vi "parsePlayInfo.vi"(7 "action":T3, 11 "variantInfo":variant) -> (3 "editArray":T1)   [LabVIEW 2014]
uses:
  typeDefs/parseAction.ctl
  typeDefs/editControl.ctl
  typeDefs/variantFlat.ctl
  typeDefs/labelInfo.ctl
  typeDefs/poiCommand.ctl
  typeDefs/jumpTpInfo.ctl
  typeDefs/syncInfo.ctl
  typeDefs/editViewPlay.ctl
panel:
  out "CODES":i32[][](array[numeric])
  out "Info":string
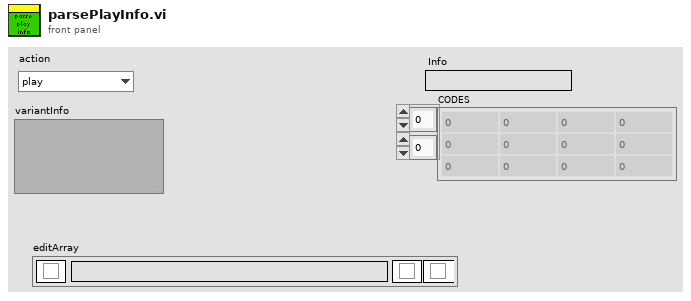
[diagram p1: front panel]
types:
  T1 = typedef "editControl.ctl" = cluster{"edit":bool, "info":string, "variantFlat":T2, "codeCluster":cluster{"code":u8[][]}, "del":bool, "ins":bool}
  T2 = typedef "variantFlat.ctl" = cluster{"type string":i16[], "data string":string}
  T3 = typedef "parseAction.ctl" = enum16{"play", "loopStart", "sync", "loopEnd", "dimm"}
  T4 = typedef "poiCommand.ctl" = u8
  T5 = typedef "labelInfo.ctl" = cluster{"LoopID":u8, "active":bool, "LoopCount":u8}
  T6 = typedef "jumpTpInfo.ctl" = cluster{"LoopID":u8, "active":bool}
  T7 = typedef "syncInfo.ctl" = cluster{"Sync-Point":u8, "active":bool}
  T8 = typedef "editViewPlay.ctl" = cluster{"delay":u16, "fromFrame":u8, "active":bool, "picIndex":i32, "toFrame":u8, "loops":u16}
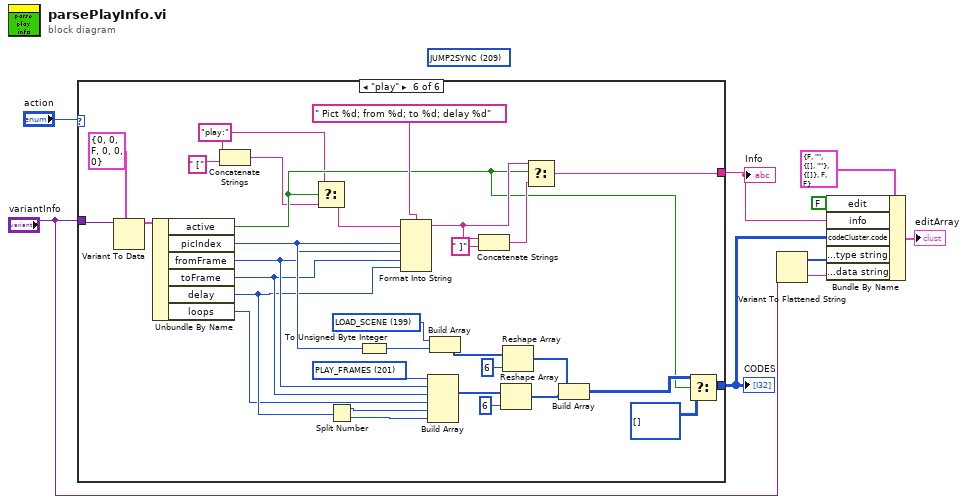
[diagram p0: block diagram]
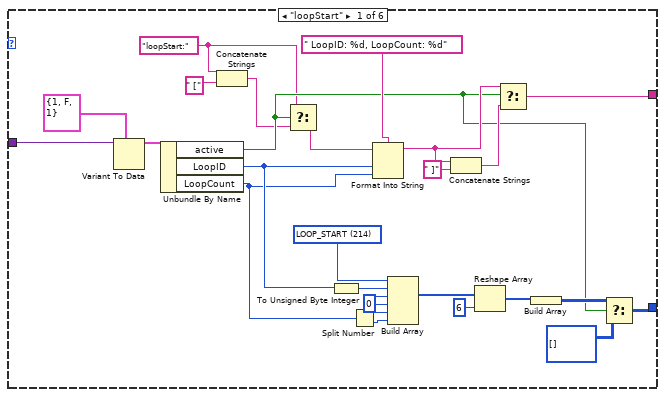
[diagram p2: hidden frame]
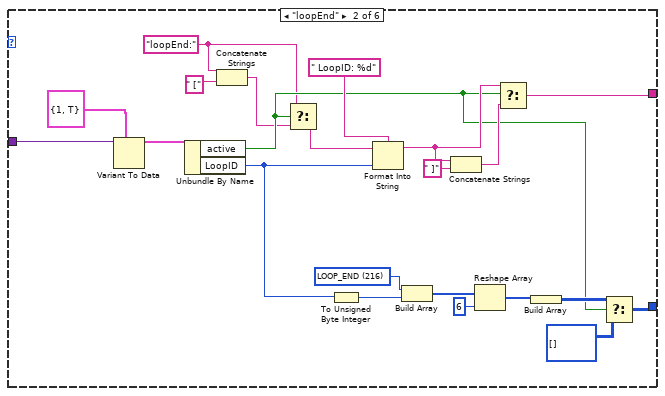
[diagram p3: hidden frame]
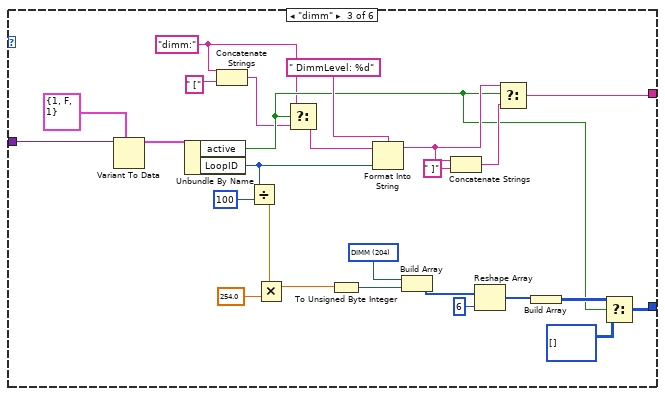
[diagram p4: hidden frame]
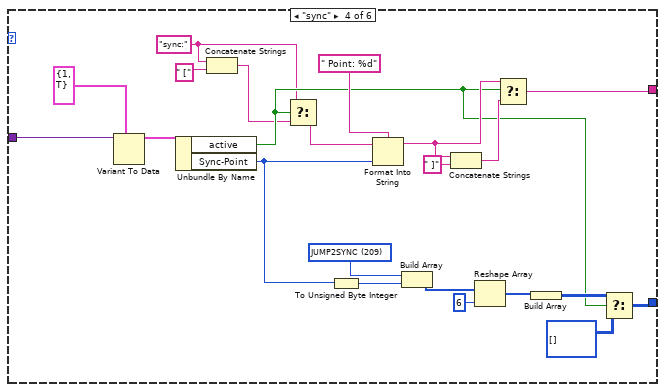
[diagram p5: hidden frame]
diagram:
  (unwired) T4 209 items=["SET_PIXEL"=0, "HEAD_SCENE"=192, "TAIL_SCENE"=193, "SAVE_SCENE"=194, "HEAD_PROG"=195, "TAIL_PROG"=196, "SAVE_PROG"=197, "INIT_FLASH"=198, "LOAD_SCENE"=199, "SHOW_RGB"=200, "PLAY_FRAMES"=201, "ANIMATE"=202, "DISPLAY_IP"=203, "DIMM"=204, "FADE2FRAME"=205, "START_PROG"=206, "STOP_PROC"=207, "PAUSE_PROC"=208, "JUMP2SYNC"=209, "CONNECT"=210, "DISCONNECT"=211, "CLIENT_DISCON"=212, "USE_SSID"=213, "LOOP_START"=214, "SYNC_POINT"=215, "LOOP_END"=216] ("Ring")
  n1 = case shown="\"play\"" "action" {
    tunnel: [w18 w41 w66 w89 _ w137] -> w6
    tunnel: [w23 w45 w71 w93 _ w118] -> w5
    tunnel: "variantInfo" -> [w19 w42 w67 w90 _ w112]
    frame "loopStart" {
      w11 = u8 0 ("unsigned 8bit integer")
      w12 = T4 214 items=["SET_PIXEL"=0, "HEAD_SCENE"=192, "TAIL_SCENE"=193, "SAVE_SCENE"=194, "HEAD_PROG"=195, "TAIL_PROG"=196, "SAVE_PROG"=197, "INIT_FLASH"=198, "LOAD_SCENE"=199, "SHOW_RGB"=200, "PLAY_FRAMES"=201, "ANIMATE"=202, "DISPLAY_IP"=203, "FADE2RGB"=204, "FADE2FRAME"=205, "START_PROG"=206, "STOP_PROC"=207, "PAUSE_PROC"=208, "JUMP2SYNC"=209, "CONNECT"=210, "DISCONNECT"=211, "CLIENT_DISCON"=212, "USE_SSID"=213, "LOOP_START"=214, "SYNC_POINT"=215, "LOOP_END"=216] ("Ring")
      w16 = "loopStart:" ("info")
      n2 = Variant To Data(type=T5 {"LoopID"=1, "active"=FALSE, "LoopCount"=1} ("labelInfo"), Variant=w19) -> (data=w20:T5)  [unwired: 1 in, 1 out]
      n3 = Unbundle By Name(w20) -> ("active"=w26:bool, "LoopID"=w22:u8, "LoopCount"=w10:u8)
      n4 = Concatenate Strings(w16, " [" ("info")) -> (w15:string)
      n5 = Select(t=w16, s=w26, f=w15) -> (s? t:f=w32:string)
      n6 = To Unsigned Byte Integer(number=w22) -> (unsigned 8bit integer=w24:u8)
      n7 = Split Number(x=w10) -> (hi(x)=w14:u8, lo(x)=w13:u8)
      n8 = Format Into String(format string=" LoopID: %d, LoopCount: %d" ("info"), initial string=w32, w22, w10) -> (resulting string=w35:string)  [unwired: 1 in, 1 out]
      n9 = Build Array(w12, w24, w11, w11, w14, w13) -> (w30:T4[])
      n10 = Concatenate Strings(w35, " ]" ("string")) -> (w34:string)
      n11 = Reshape Array(w30, 6 ("dimension size")) -> (w28:T4[])
      n12 = Select(t=w35, s=w26, f=w34) -> (s? t:f=w18:string)
      n13 = Build Array(w28) -> (w27:T4[][])
      n14 = Select(t=w27, s=w26, f=i32[][] []) -> (s? t:f=w23:i32[][])
    }
    frame "loopEnd" {
      w37 = T4 216 items=["SET_PIXEL"=0, "HEAD_SCENE"=192, "TAIL_SCENE"=193, "SAVE_SCENE"=194, "HEAD_PROG"=195, "TAIL_PROG"=196, "SAVE_PROG"=197, "INIT_FLASH"=198, "LOAD_SCENE"=199, "SHOW_RGB"=200, "PLAY_FRAMES"=201, "ANIMATE"=202, "DISPLAY_IP"=203, "FADE2RGB"=204, "FADE2FRAME"=205, "START_PROG"=206, "STOP_PROC"=207, "PAUSE_PROC"=208, "JUMP2SYNC"=209, "CONNECT"=210, "DISCONNECT"=211, "CLIENT_DISCON"=212, "USE_SSID"=213, "LOOP_START"=214, "SYNC_POINT"=215, "LOOP_END"=216] ("Ring")
      w39 = "loopEnd:" ("info")
      n15 = Variant To Data(type=T6 {"LoopID"=1, "active"=TRUE} ("jumptoInfo"), Variant=w42) -> (data=w43:T6)  [unwired: 1 in, 1 out]
      n16 = Unbundle By Name(w43) -> ("active"=w48:bool, "LoopID"=w44:u8)
      n17 = Concatenate Strings(w39, " [" ("info")) -> (w38:string)
      n18 = Select(t=w39, s=w48, f=w38) -> (s? t:f=w54:string)
      n19 = To Unsigned Byte Integer(number=w44) -> (unsigned 8bit integer=w46:u8)
      n20 = Format Into String(format string=" LoopID: %d" ("info"), initial string=w54, w44) -> (resulting string=w57:string)  [unwired: 1 in, 1 out]
      n21 = Build Array(w37, w46) -> (w52:T4[])
      n22 = Concatenate Strings(w57, " ]" ("string")) -> (w56:string)
      n23 = Reshape Array(w52, 6 ("dimension size")) -> (w50:T4[])
      n24 = Select(t=w57, s=w48, f=w56) -> (s? t:f=w41:string)
      n25 = Build Array(w50) -> (w49:T4[][])
      n26 = Select(t=w49, s=w48, f=i32[][] []) -> (s? t:f=w45:i32[][])
    }
    frame "dimm" {
      w58 = T4 204 items=["SET_PIXEL"=0, "HEAD_SCENE"=192, "TAIL_SCENE"=193, "SAVE_SCENE"=194, "HEAD_PROG"=195, "TAIL_PROG"=196, "SAVE_PROG"=197, "INIT_FLASH"=198, "LOAD_SCENE"=199, "SHOW_RGB"=200, "PLAY_FRAMES"=201, "ANIMATE"=202, "DISPLAY_IP"=203, "DIMM"=204, "FADE2FRAME"=205, "START_PROG"=206, "STOP_PROC"=207, "PAUSE_PROC"=208, "JUMP2SYNC"=209, "CONNECT"=210, "DISCONNECT"=211, "CLIENT_DISCON"=212, "USE_SSID"=213, "LOOP_START"=214, "SYNC_POINT"=215, "LOOP_END"=216] ("Ring")
      w64 = "dimm:" ("info")
      n27 = Variant To Data(type=T5 {"LoopID"=1, "active"=FALSE, "LoopCount"=1} ("labelInfo"), Variant=w67) -> (data=w68:T5)  [unwired: 1 in, 1 out]
      n28 = Unbundle By Name(w68) -> ("active"=w74:bool, "LoopID"=w70:u8)
      n29 = Concatenate Strings(w64, " [" ("info")) -> (w63:string)
      n30 = Divide(x=w70, y=u8 100) -> (x/y=w61:dbl)
      n31 = Multiply(x=w61, y=254.0) -> (x*y=w62:dbl)
      n32 = Select(t=w64, s=w74, f=w63) -> (s? t:f=w80:string)
      n33 = To Unsigned Byte Integer(number=w62) -> (unsigned 8bit integer=w72:u8)
      n34 = Format Into String(format string=" DimmLevel: %d" ("info"), initial string=w80, w70) -> (resulting string=w83:string)  [unwired: 1 in, 1 out]
      n35 = Build Array(w58, w72) -> (w78:T4[])
      n36 = Concatenate Strings(w83, " ]" ("string")) -> (w82:string)
      n37 = Reshape Array(w78, 6 ("dimension size")) -> (w76:T4[])
      n38 = Select(t=w83, s=w74, f=w82) -> (s? t:f=w66:string)
      n39 = Build Array(w76) -> (w75:T4[][])
      n40 = Select(t=w75, s=w74, f=i32[][] []) -> (s? t:f=w71:i32[][])
    }
    frame "sync" {
      w84 = T4 209 items=["SET_PIXEL"=0, "HEAD_SCENE"=192, "TAIL_SCENE"=193, "SAVE_SCENE"=194, "HEAD_PROG"=195, "TAIL_PROG"=196, "SAVE_PROG"=197, "INIT_FLASH"=198, "LOAD_SCENE"=199, "SHOW_RGB"=200, "PLAY_FRAMES"=201, "ANIMATE"=202, "DISPLAY_IP"=203, "DIMM"=204, "FADE2FRAME"=205, "START_PROG"=206, "STOP_PROC"=207, "PAUSE_PROC"=208, "JUMP2SYNC"=209, "CONNECT"=210, "DISCONNECT"=211, "CLIENT_DISCON"=212, "USE_SSID"=213, "LOOP_START"=214, "SYNC_POINT"=215, "LOOP_END"=216] ("Ring")
      w88 = "sync:" ("info")
      n41 = Variant To Data(type=T7 {"Sync-Point"=1, "active"=TRUE} ("syncInfo"), Variant=w90) -> (data=w91:T7)  [unwired: 1 in, 1 out]
      n42 = Unbundle By Name(w91) -> ("active"=w96:bool, "Sync-Point"=w92:u8)
      n43 = Concatenate Strings(w88, " [" ("info")) -> (w87:string)
      n44 = Select(t=w88, s=w96, f=w87) -> (s? t:f=w102:string)
      n45 = To Unsigned Byte Integer(number=w92) -> (unsigned 8bit integer=w94:u8)
      n46 = Format Into String(format string=" Point: %d" ("info"), initial string=w102, w92) -> (resulting string=w105:string)  [unwired: 1 in, 1 out]
      n47 = Build Array(w84, w94) -> (w100:T4[])
      n48 = Concatenate Strings(w105, " ]" ("string")) -> (w104:string)
      n49 = Reshape Array(w100, 6 ("dimension size")) -> (w98:T4[])
      n50 = Select(t=w105, s=w96, f=w104) -> (s? t:f=w89:string)
      n51 = Build Array(w98) -> (w97:T4[][])
      n52 = Select(t=w97, s=w96, f=i32[][] []) -> (s? t:f=w93:i32[][])
    }
    frame Default {
    }
    frame "play" {
      w106 = T4 201 items=["SET_PIXEL"=0, "HEAD_SCENE"=192, "TAIL_SCENE"=193, "SAVE_SCENE"=194, "HEAD_PROG"=195, "TAIL_PROG"=196, "SAVE_PROG"=197, "INIT_FLASH"=198, "LOAD_SCENE"=199, "SHOW_RGB"=200, "PLAY_FRAMES"=201, "ANIMATE"=202, "DISPLAY_IP"=203, "FADE2RGB"=204, "FADE2FRAME"=205, "START_PROG"=206, "STOP_PROC"=207, "PAUSE_PROC"=208, "JUMP2SYNC"=209, "CONNECT"=210, "DISCONNECT"=211, "CLIENT_DISCON"=212, "USE_SSID"=213, "LABEL"=214, "SYNC_POINT"=215, "LOOP"=216] ("Ring")
      w107 = T4 199 items=["SET_PIXEL"=0, "HEAD_SCENE"=192, "TAIL_SCENE"=193, "SAVE_SCENE"=194, "HEAD_PROG"=195, "TAIL_PROG"=196, "SAVE_PROG"=197, "INIT_FLASH"=198, "LOAD_SCENE"=199, "SHOW_RGB"=200, "PLAY_FRAMES"=201, "ANIMATE"=202, "DISPLAY_IP"=203, "FADE2RGB"=204, "FADE2FRAME"=205, "START_PROG"=206, "STOP_PROC"=207, "PAUSE_PROC"=208, "JUMP2SYNC"=209, "CONNECT"=210, "DISCONNECT"=211, "CLIENT_DISCON"=212, "USE_SSID"=213, "LABEL"=214, "SYNC_POINT"=215, "LOOP"=216] ("Ring")
      w110 = "play:" ("info")
      n53 = Variant To Data(type=T8 {"delay"=0, "fromFrame"=0, "active"=FALSE, "picIndex"=0, "toFrame"=0, "loops"=0} ("editDefPlay"), Variant=w112) -> (data=w113:T8)  [unwired: 1 in, 1 out]
      n54 = Unbundle By Name(w113) -> ("active"=w117:bool, "picIndex"=w131:i32, "fromFrame"=w124:u8, "toFrame"=w123:u8, "delay"=w122:u16, "loops"=w108:u16)
      n55 = Concatenate Strings(w110, " [" ("info")) -> (w109:string)
      n56 = Select(t=w110, s=w117, f=w109) -> (s? t:f=w133:string)
      n57 = Split Number(x=w122) -> (hi(x)=w121:u8, lo(x)=w120:u8)
      n58 = To Unsigned Byte Integer(number=w131) -> (unsigned 8bit integer=w115:u8)
      n59 = Format Into String(format string=" Pict %d; from %d; to %d; delay %d" ("info"), initial string=w133, w131, w124, w123, w122) -> (resulting string=w136:string)  [unwired: 1 in, 1 out]
      n60 = Build Array(w106, w124, w123, w108, w121, w120) -> (w127:u16[])
      n61 = Build Array(w107, w115) -> (w130:T4[])
      n62 = Concatenate Strings(w136, " ]" ("string")) -> (w135:string)
      n63 = Reshape Array(w127, 6 ("dimension size")) -> (w125:u16[])
      n64 = Reshape Array(w130, 6 ("dimension size")) -> (w126:T4[])
      n65 = Select(t=w136, s=w117, f=w135) -> (s? t:f=w137:string)
      n66 = Build Array(w126, w125) -> (w119:u16[][])
      n67 = Select(t=w119, s=w117, f=i32[][] []) -> (s? t:f=w118:i32[][])
    }
  }
  "Info" <- w6
  "CODES" <- w5
  n68 = Variant To Flattened String(Variant="variantInfo") -> (data string=w2:string, 1:w3:i16[])
  n69 = Bundle By Name(cluster=T1 {"edit"=FALSE, "info"="", "variantFlat"={"type string"=[], "data string"=""}, "codeCluster"={"code"=[]}, "del"=FALSE, "ins"=FALSE} ("editCntrl"), "edit"=FALSE, "info"=w6, "codeCluster.code"=w5, "variantFlat.type string"=w3, "variantFlat.data string"=w2) -> (→"editArray":T1)
